vi "HovaCAL Stufentabelle aendern.vi"(8 "Fehler (Eingang, kein Fehler)":errorcluster, 10 "TestKonfig alt":T1 {"TestKonfig Interferent"."Gasflasche MFC3" items=["----"=10000, "IAG NH3 3000"=0, "IAG NH3 200"=1, "IAG NH3 2000"=2, "IAG MG"=3, "IAG O2"=4]; "TestKonfig Interferent"."Gasflasche MFC2" items=["----"=10000, "IAG NH3 3000"=0, "IAG NH3 200"=1, "IAG NH3 2000"=2, "IAG MG"=3, "IAG O2"=4]; "TestKonfig Interferent"."Eingangs Konzentration MFC1" min=0.0; "TestKonfig Interferent"."Ausgangs Konzentration MFC1" min=0.0; "TestKonfig Interferent"."MFC2" items=["MFC 2", "MFC 3", "MFC 4", "MFC 5"]; "TestKonfig Interferent"."MFC3" items=["MFC 2", "MFC 3", "MFC 4", "MFC 5"]; "TestKonfig Interferent"."Ausgangs Konzentration MFC3" min=0.0; "TestKonfig Interferent"."Eingangs Konzentration MFC3" min=0.0; "TestKonfig Interferent"."Ausgangs Konzentration MFC2" min=0.0; "TestKonfig Interferent"."Eingangs Konzentration MFC2" min=0.0; "TestKonfig H2O"."HovaCAL Temperature" format="%.2f"; "TestKonfig H2O"."HovaCAL Flow Input Cluster"."HovaCAL Flow Input Cluster" format="%.2f"; "TestKonfig H2O"."Eingangs Konzentration:" min=0.0; "TestKonfig H2O"."zusätzliche Zeitdauer Erster Punkt" min=30 step=1 format="%#_5g"; "TestKonfig H2O"."Zeitdauer Stufen" format="%#_5g"; "TestKonfig H2O"."Max Fehler" format="%#_5g"; "TestKonfig H2O"."Anzahl Stufen" format="%#_5g"; "TestKonfig H2O"."Modus" items=["Messen", "CG zu Entnahmestelle"]}, 11 "TestKonfig (Eingang)":T1 {"TestKonfig Interferent"."Gasflasche MFC3" items=["----"=10000, "IAG NH3 3000"=0, "IAG NH3 200"=1, "IAG NH3 2000"=2, "IAG MG"=3, "IAG O2"=4]; "TestKonfig Interferent"."Gasflasche MFC2" items=["----"=10000, "IAG NH3 3000"=0, "IAG NH3 200"=1, "IAG NH3 2000"=2, "IAG MG"=3, "IAG O2"=4]; "TestKonfig Interferent"."Eingangs Konzentration MFC1" min=0.0; "TestKonfig Interferent"."Ausgangs Konzentration MFC1" min=0.0; "TestKonfig Interferent"."MFC2" items=["MFC 2", "MFC 3", "MFC 4", "MFC 5"]; "TestKonfig Interferent"."MFC3" items=["MFC 2", "MFC 3", "MFC 4", "MFC 5"]; "TestKonfig Interferent"."Ausgangs Konzentration MFC3" min=0.0; "TestKonfig Interferent"."Eingangs Konzentration MFC3" min=0.0; "TestKonfig Interferent"."Ausgangs Konzentration MFC2" min=0.0; "TestKonfig Interferent"."Eingangs Konzentration MFC2" min=0.0; "TestKonfig H2O"."HovaCAL Temperature" format="%.2f"; "TestKonfig H2O"."HovaCAL Flow Input Cluster"."HovaCAL Flow Input Cluster" format="%.2f"; "TestKonfig H2O"."Eingangs Konzentration:" min=0.0; "TestKonfig H2O"."zusätzliche Zeitdauer Erster Punkt" min=30 step=1 format="%#_5g"; "TestKonfig H2O"."Zeitdauer Stufen" format="%#_5g"; "TestKonfig H2O"."Max Fehler" format="%#_5g"; "TestKonfig H2O"."Anzahl Stufen" format="%#_5g"; "TestKonfig H2O"."Modus" items=["Messen", "CG zu Entnahmestelle"]}) -> (0 "Fehler (Ausgang)":errorcluster, 3 "TestKonfig (Ausgang)":T1 {"TestKonfig Interferent"."Gasflasche MFC3" items=["----"=10000, "IAG NH3 3000"=0, "IAG NH3 200"=1, "IAG NH3 2000"=2, "IAG MG"=3, "IAG O2"=4]; "TestKonfig Interferent"."Gasflasche MFC2" items=["----"=10000, "IAG NH3 3000"=0, "IAG NH3 200"=1, "IAG NH3 2000"=2, "IAG MG"=3, "IAG O2"=4]; "TestKonfig Interferent"."Eingangs Konzentration MFC1" min=0.0; "TestKonfig Interferent"."Ausgangs Konzentration MFC1" min=0.0; "TestKonfig Interferent"."MFC2" items=["MFC 2", "MFC 3", "MFC 4", "MFC 5"]; "TestKonfig Interferent"."MFC3" items=["MFC 2", "MFC 3", "MFC 4", "MFC 5"]; "TestKonfig Interferent"."Ausgangs Konzentration MFC3" min=0.0; "TestKonfig Interferent"."Eingangs Konzentration MFC3" min=0.0; "TestKonfig Interferent"."Ausgangs Konzentration MFC2" min=0.0; "TestKonfig Interferent"."Eingangs Konzentration MFC2" min=0.0; "TestKonfig H2O"."HovaCAL Temperature" format="%.2f"; "TestKonfig H2O"."HovaCAL Flow Input Cluster"."HovaCAL Flow Input Cluster" format="%.2f"; "TestKonfig H2O"."Eingangs Konzentration:" min=0.0; "TestKonfig H2O"."zusätzliche Zeitdauer Erster Punkt" min=30 step=1 format="%#_5g"; "TestKonfig H2O"."Zeitdauer Stufen" format="%#_5g"; "TestKonfig H2O"."Max Fehler" format="%#_5g"; "TestKonfig H2O"."Anzahl Stufen" format="%#_5g"; "TestKonfig H2O"."Modus" items=["Messen", "CG zu Entnahmestelle"]})   [LabVIEW 2020, in "EPA 1065.lvlib" / "HovaCAL Interference verificaton.lvlib"]
uses:
  HovaCAL Interference verificaton.lvlib
  TestKonfig.ctl
  TestKonfig H2O.ctl
  Modus.ctl
  Linearisierung V2/SpanEinstellungen/Einheit.ctl
  Linearisierung V2/Gasteiler/Stufen Tabelle.ctl
  Linearisierung V2/Gasteiler/HovaCAL_Interface/Controls/Flow Einstellung.ctl
  Linearisierung V2/Gasteiler/HovaCAL_Interface/Controls/Temp Sollwerte Anzeige.ctl
  TestKonfig Interferents.ctl
  MFCAuswahl.ctl
  Seiten/System Einstellungen V2/Gasflasche Auswahl.ctl
  Linearisierung V2/Gasteiler/Aktionen FGV Gasteiler Daten.ctl
  Linearisierung V2/Gasteiler/HovaCal/HovaCal.lvlib
  Linearisierung V2/Gasteiler/Gasteiler.lvlib
  Linearisierung V2/SpanEinstellungen/SpanEinstellungen.lvlib
  Linearisierung V2/Gasteiler/HovaCAL_Interface/Controls/Controls.lvlib
  Seiten/System Einstellungen V2/System Einstellungen V2.lvlib
panel:
  # "sec"
  # "%"
  # "sec"
  # "sec"
  # "%"
  # "sec"
  # "sec"
  # "%"
  # "sec"
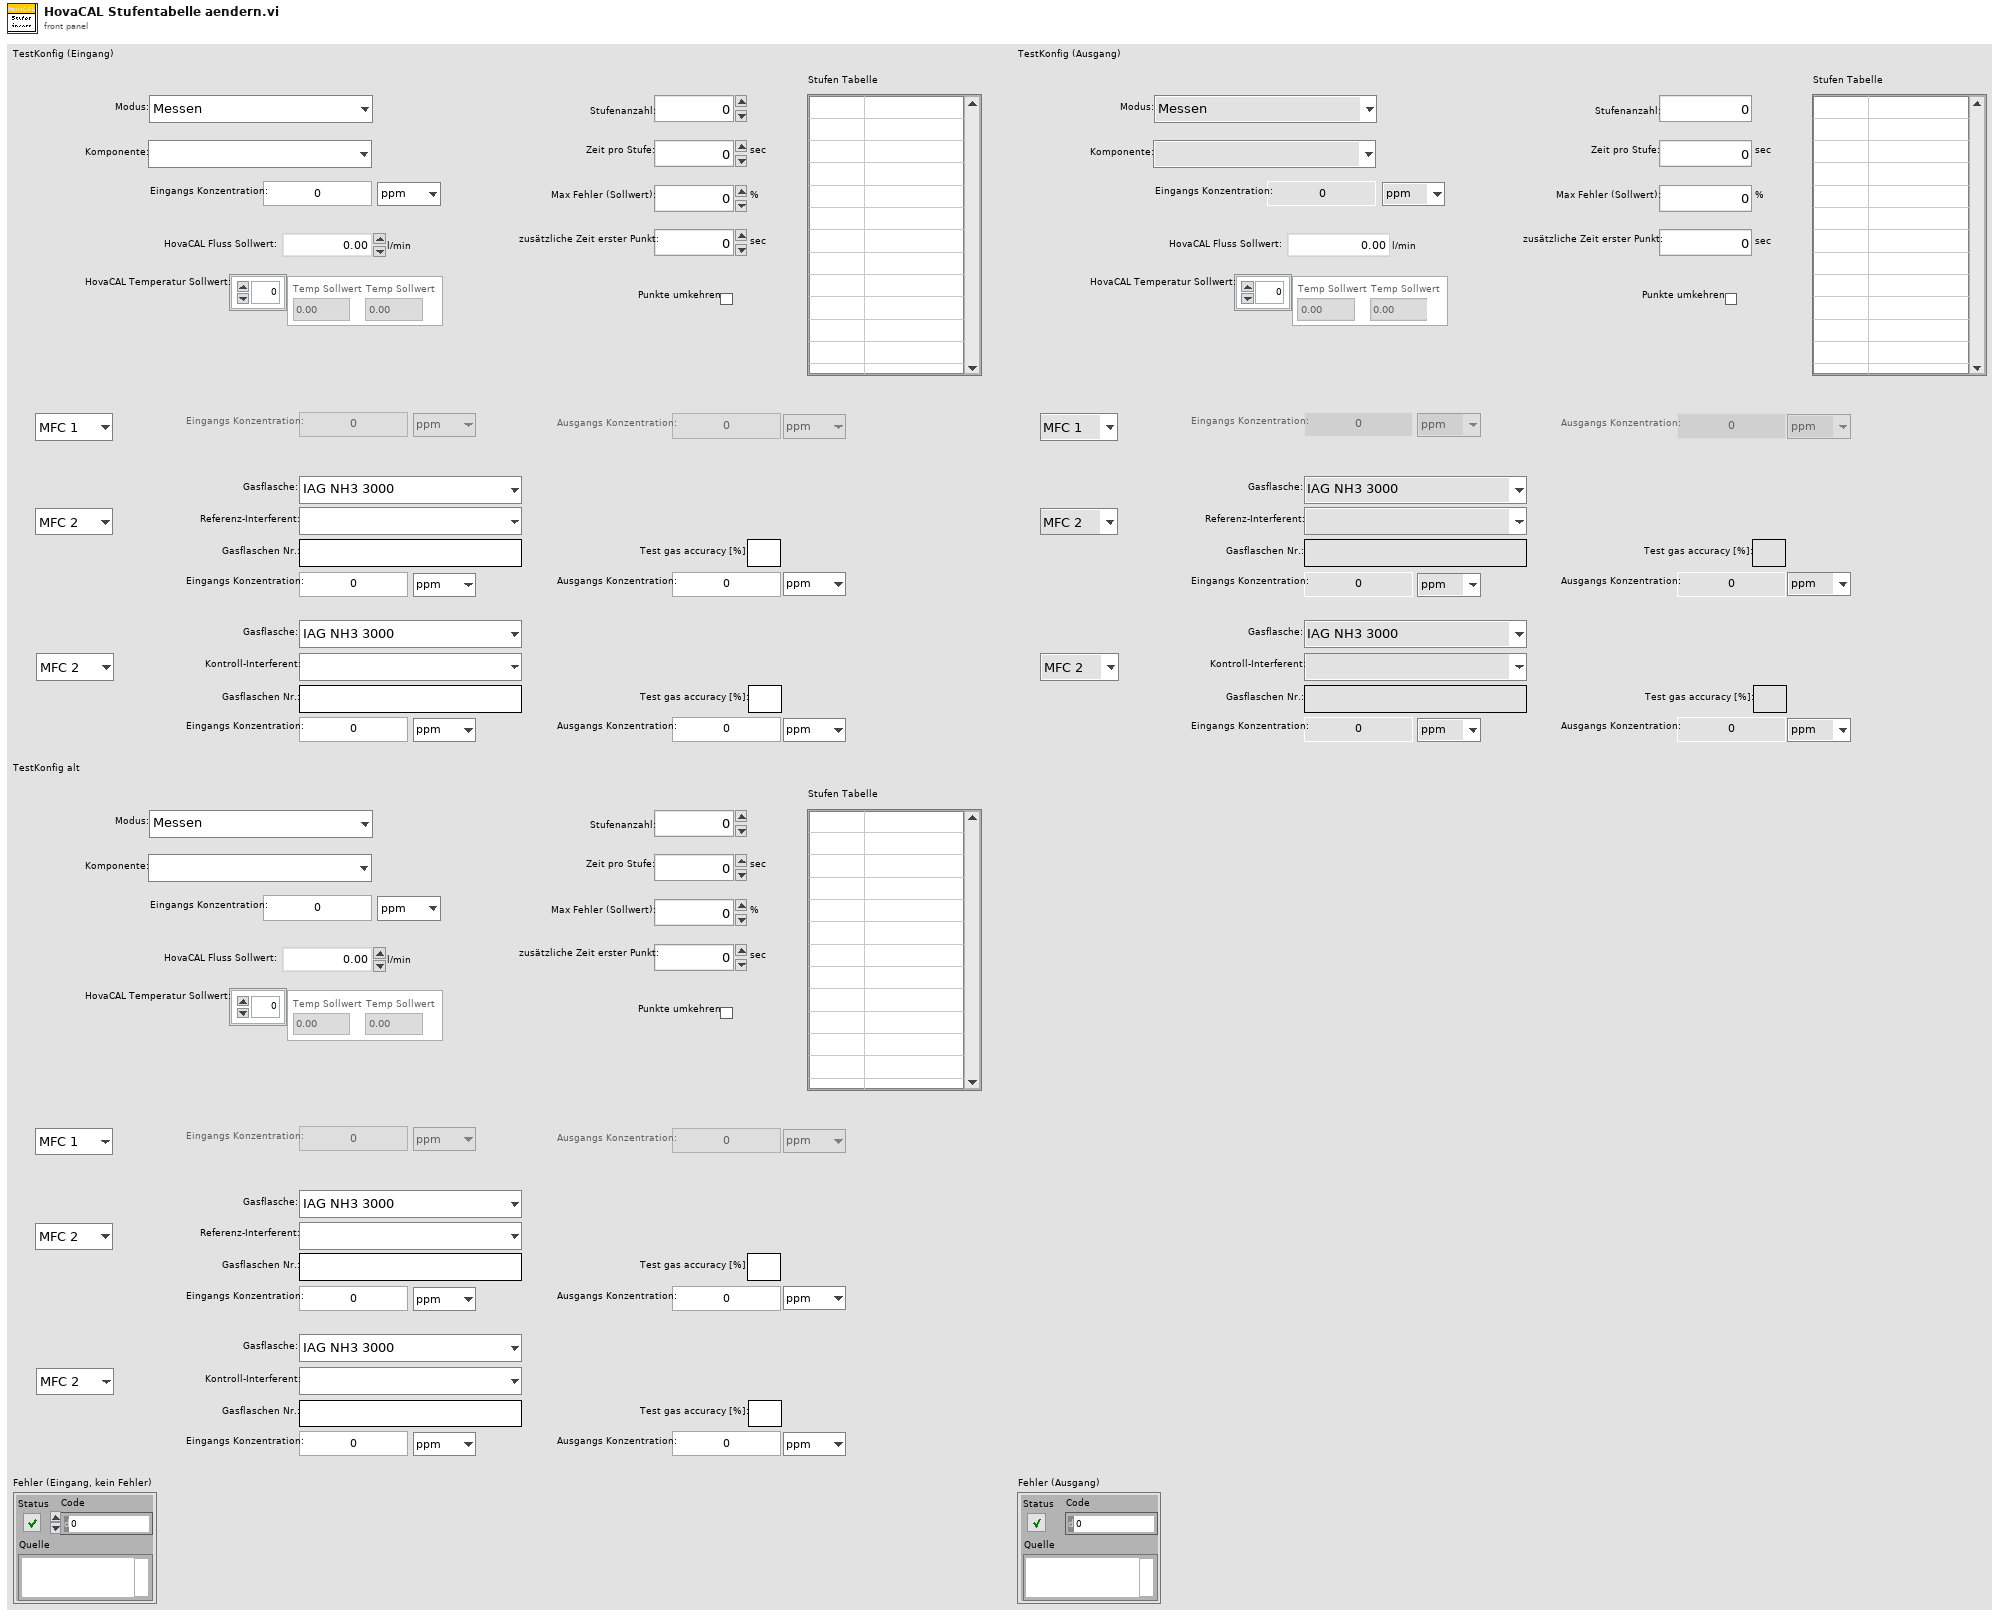
[diagram p1: front panel]
types:
  T1 = typedef "EPA 1065.lvlib/HovaCAL Interference verificaton.lvlib/TestKonfig.ctl" = cluster{"TestKonfig H2O":T2, "TestKonfig Interferent":T8}
  T2 = typedef "EPA 1065.lvlib/HovaCAL Interference verificaton.lvlib/TestKonfig H2O.ctl" = cluster{"Modus":T3, "Komponente:":u16, "Eingangs Konzentration:":dbl, "Einheit":T4, "Anzahl Stufen":sgl, "Zeitdauer Stufen":sgl, "Max Fehler":sgl, "zusätzliche Zeitdauer Erster Punkt":sgl, "Punkte umkehren":bool, "Stufen Tabelle":T5, "HovaCAL Flow Input Cluster":T6, "HovaCAL Temperature":T7}
  T3 = typedef "EPA 1065.lvlib/HovaCAL Interference verificaton.lvlib/Modus.ctl" = u16
  T4 = typedef "Linearisierung v2.lvlib/SpanEinstellungen.lvlib/Einheit.ctl" = enum16{"ppm", "%"}
  T5 = typedef "Linearisierung v2.lvlib/Gasteiler.lvlib/Stufen Tabelle.ctl" = string[][]
  T6 = typedef "Linearisierung v2.lvlib/Gasteiler.lvlib/HovaCAL_Interface.lvlib/Controls.lvlib/Flow Einstellung.ctl" = cluster{"HovaCAL Flow Input Cluster":dbl}
  T7 = typedef "Linearisierung v2.lvlib/Gasteiler.lvlib/HovaCAL_Interface.lvlib/Controls.lvlib/Temp Sollwerte Anzeige.ctl" = dbl[]
  T8 = typedef "EPA 1065.lvlib/HovaCAL Interference verificaton.lvlib/TestKonfig Interferents.ctl" = cluster{"MFC1":enum16{"MFC 1"}, "Eingangs Konzentration MFC1":dbl, "Einheit MFC1 Eingang":T4, "Ausgangs Konzentration MFC1":dbl, "Einheit MFC1 Ausgang":T4, "MFC2":T9, "Referenz-Interferent:":u16, "Gasflaschen Nr MFC2":string, "Eingangs Konzentration MFC2":dbl, "Einheit MFC2 Eingang":T4, "Accuracy MFC2":string, "Ausgangs Konzentration MFC2":dbl, "Einheit MFC2 Ausgang":T4, "MFC3":T9, "Kontroll-Interferent:":u16, "Gasflaschen Nr MFC3":string, "Accuracy MFC3":string, "Eingangs Konzentration MFC3":dbl, "Einheit MFC3 Eingang":T4, "Ausgangs Konzentration MFC3":dbl, "Einheit MFC3 Ausgang":T4, "Gasflasche MFC2":T10, "Gasflasche MFC3":T10}
  T9 = typedef "EPA 1065.lvlib/HovaCAL Interference verificaton.lvlib/MFCAuswahl.ctl" = u16
  T10 = typedef "System Einstellungen V2.lvlib/Gasflasche Auswahl.ctl" = u16
  T11 = typedef "Linearisierung v2.lvlib/Gasteiler.lvlib/Aktionen FGV Gasteiler Daten.ctl" = enum16{"lesen", "Gasteiler Daten", "Seriellen Param.", "MB-Endwert", "laden", "speichern", "Anforderung", "TCP", "Aufzeichnung Start"}
  T12 = typedef "Linearisierung v2.lvlib/Gasteiler.lvlib/Gasteiler Daten.ctl" = cluster{"Gasteiler":T13, "Gasteiler Stufen":T14, "Gasteiler Type":T15, "Konfig Gasteiler":T16, "Gasteiler Span Eingänge":u16}
  T13 = typedef "String - Eingabefeld.ctl" = string
  T14 = typedef "Linearisierung v2.lvlib/Gasteiler.lvlib/Gasteiler Stufen.ctl" = u16
  T15 = typedef "Linearisierung v2.lvlib/GasteilerType.ctl" = u16
  T16 = typedef "System Einstellungen V2.lvlib/Gasteiler Auswahl.ctl" = u16
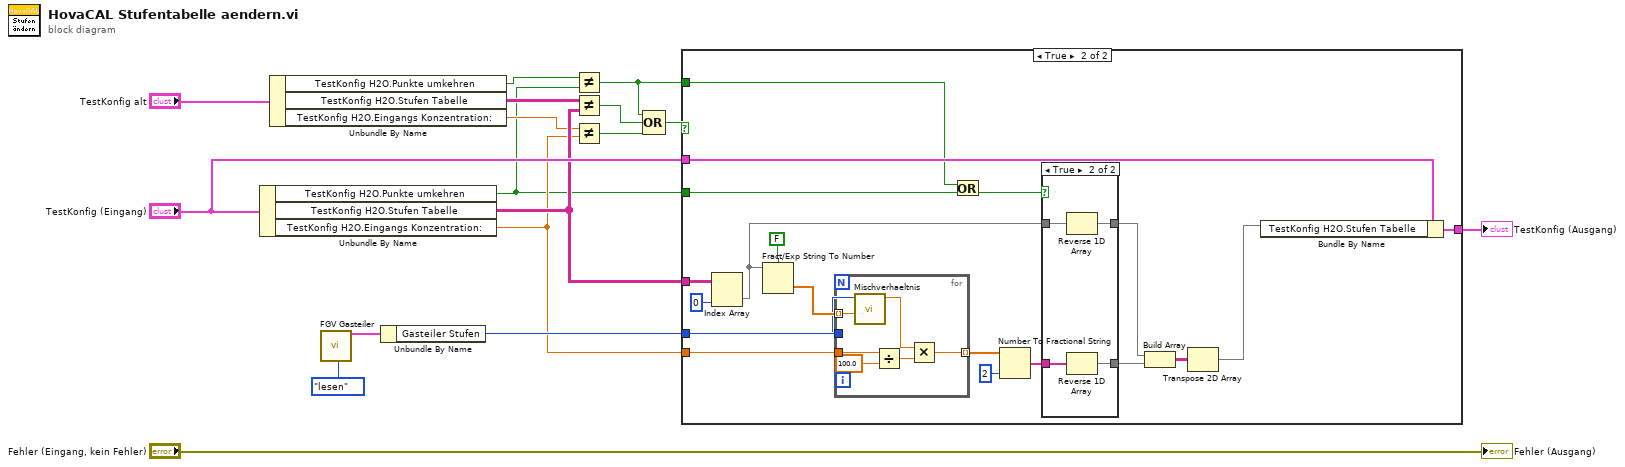
[diagram p0: block diagram]
diagram:
  n1 = Unbundle By Name("TestKonfig (Eingang)") -> ("TestKonfig H2O.Punkte umkehren"=w2:bool, "TestKonfig H2O.Stufen Tabelle"=w10:T5, "TestKonfig H2O.Eingangs Konzentration:"=w8:dbl)
  n2 = Unbundle By Name("TestKonfig alt") -> ("TestKonfig H2O.Punkte umkehren"=w3:bool, "TestKonfig H2O.Stufen Tabelle"=w11:T5, "TestKonfig H2O.Eingangs Konzentration:"=w9:dbl)
  n3 = call "FGV Gasteiler.vi"("Aktionen"=Aktionen_FGV_Gasteiler_Daten."lesen") -> ("Gasteiler Daten"=w14:T12)  [unwired: 11 in, 7 out]
  n4 = Unbundle By Name(w14) -> ("Gasteiler Stufen"=w15:T14)
  n5 = Not Equal?(x=w3, y=w2) -> (x != y?=w1:bool)
  n6 = Not Equal?(x=w11, y=w10) -> (x != y?=w7:bool)
  n7 = Not Equal?(x=w9, y=w8) -> (x != y?=w6:bool)
  n8 = Compound Arithmetic op=OR ("Mehrfacharithmetik")(w1, w7, w6) -> (w4:bool)
  n9 = case shown="True" w4 {
    tunnel: "TestKonfig (Eingang)" -> [w18 w37]
    tunnel: [w18 w36] -> w16
    tunnel: w15 -> [_ w33]
    tunnel: w10 -> [_ w28]
    tunnel: w8 -> [_ w27]
    tunnel: w2 -> [_ w26]
    tunnel: w1 -> [_ w19]
    frame False {
    }
    frame True {
      n10 = Index Array(array=w28, index (col)=0 ("Deaktivierter Index (Spalte)")) -> (element=w25:string[])  [unwired: 1 in]
      n11 = Fract/Exp String To Number(use system decimal point (T)=FALSE ("Systemdezimalzeichen verwenden (T)"), string=w25) -> (number=w30:dbl[])  [unwired: 2 in, 1 out]
      n12 = for {
        tunnel: w30 -> [w49] mode=indexing
        tunnel: w33 -> [w50]
        tunnel: w27 -> [w48]
        tunnel: [w44] -> w31 mode=indexing
        n13 = call "Mischverhaeltnis.vi"("Konzentration"=w49, "Sollwert"=w50) -> ("%"=w45:dbl)  [unwired: 8 in, 1 out]
        n14 = Divide(x=w48, y=sgl 100.0) -> (x/y=w46:dbl)
        n15 = Multiply(x=w45, y=w46) -> (x*y=w44:dbl)
      }
      n16 = Or(x=w19, y=w26) -> (x .or. y?=w20:bool)
      n17 = Number To Fractional String(number=w31, precision (6)=i16 2 ("Genauigkeit (6)")) -> (F-format string=w24:string[])  [unwired: 2 in]
      n18 = case shown="True" w20 {
        tunnel: w25 -> [w39 w43]
        tunnel: w24 -> [w38 w42]
        tunnel: [w38 w41] -> w23
        tunnel: [w39 w40] -> w22
        frame False {
        }
        frame True {
          n19 = Reverse 1D Array(array=w43) -> (reversed array=w40:string[])
          n20 = Reverse 1D Array(array=w42) -> (reversed array=w41:string[])
        }
      }
      n21 = Build Array(w22, w23) -> (w35:string[][])
      n22 = Transpose 2D Array(2D array=w35) -> (transposed array=w21:string[][])
      n23 = Bundle By Name(cluster=w37, "TestKonfig H2O.Stufen Tabelle"=w21) -> (w36:T1)
    }
  }
  "TestKonfig (Ausgang)" <- w16
  "Fehler (Ausgang)" <- "Fehler (Eingang, kein Fehler)"
